vi "Lab Panel V4.91.vi"() -> ()   [LabVIEW 2013] (continued)
                            n840 = call "Save data file (stop) v3.vi"("panel id"=w1524) -> ("network file save error"=w1523:errorcluster)  [unwired: 9 in, 1 out]
                            n841 = local write "RESULT LAB04-1"(FALSE) -> ()
                            n842 = local write "data file error"(w1523) -> ()
                          }
                        }
                        n843 = Bundle(cluster=w1520, "STATUS"="STOP") -> (w1518:T4)  [unwired: 2 in]
                        n844 = local write "DISP LAB04-1"(w1518) -> ()
                      }
                    }
                  }
                  frame True {
                    n845 = local read "SIG LAB04-1"() -> (w1527:T2)
                    n846 = stacked-sequence {
                      seq-local: [w1538 _] -> [_ w1542]
                      tunnel: w1536 -> [_ w1552]
                      tunnel: w1535 -> [_ w1551]
                      tunnel: w1534 -> [_ w1550]
                      tunnel: w1533 -> [_ w1549]
                      tunnel: w1532 -> [_ w1548]
                      tunnel: [_ w1547] -> w1531
                      tunnel: w1530 -> [_ w1546]
                      tunnel: w1529 -> [_ w1545]
                      tunnel: w1528 -> [_ w1544]
                      tunnel: w1527 -> [w1537 w1543]
                      tunnel: w1526 -> [_ w1541]
                      frame #0 {
                        n847 = Unbundle(w1537) -> ("AMPS"=w1540:dbl)  [unwired: 4 out]
                        n848 = call "Check For Amps on v1.vi"("ID"="LAB04-1", "amps"=w1540) -> ("amps"=w1538:bool)  [unwired: 9 in]
                      }
                      frame #1 {
                        n849 = case shown="True" w1542 {
                          tunnel: w1552 -> [_ w1565]
                          tunnel: w1551 -> [_ w1564]
                          tunnel: w1550 -> [_ w1563]
                          tunnel: w1549 -> [_ w1562]
                          tunnel: w1548 -> [_ w1561]
                          tunnel: [errorcluster {"status"=FALSE, "code"=0, "source"=""} ("error out") w1560] -> w1547
                          tunnel: w1546 -> [_ w1559]
                          tunnel: w1545 -> [_ w1558]
                          tunnel: w1544 -> [_ w1557]
                          tunnel: w1543 -> [_ w1556]
                          tunnel: w1541 -> [_ w1555]
                          frame False {
                            w1553 = FALSE
                            n850 = local write "RUN LAB04-1"(w1553) -> ()
                            n851 = local write "run lab04-1"(w1553) -> ()
                          }
                          frame True {
                            n852 = stacked-sequence {
                              seq-local: [w1566 _ _ _ _] -> [_ w1590 _ _ _]
                              tunnel: w1565 -> [w1571 _ _ _ _]
                              tunnel: w1564 -> [w1567 _ _ _ _]
                              tunnel: w1563 -> [w1581 _ _ _ _]
                              tunnel: w1562 -> [w1574 _ _ _ _]
                              tunnel: w1561 -> [w1569 _ _ _ _]
                              tunnel: [_ w1585 _ _ _] -> w1560
                              tunnel: w1559 -> [_ _ _ w1611 _]
                              tunnel: w1558 -> [_ _ _ w1610 _]
                              tunnel: w1557 -> [_ _ _ w1609 _]
                              tunnel: w1556 -> [_ _ _ _ _]
                              tunnel: w1555 -> [_ _ _ _ w1625]
                              frame #0 {
                                w1568 = "\\"
                                n853 = local read "SET LAB04-1"() -> (w1576:T5)
                                n854 = case shown="\"CYCLE TEST\"" w1581 {
                                tunnel: ["L04-1-CHART TEST-" "L04-1-CYCLE TEST-" "L04-1-T-RISE TEST-"] -> w1577
                                frame "CHART TEST", Default {
                                }
                                frame "CYCLE TEST" {
                                }
                                frame "T-RISE TEST" {
                                }
                                }
                                n855 = Unbundle(w1576) -> ("DESCRIPTION"=w1575:string)  [unwired: 4 out]
                                n856 = Concatenate Strings(w1571, "\\", w1569, w1568, w1567, w1568) -> (w1578:string)
                                n857 = String To Path(string=w1578) -> (path=w1580:path)
                                n858 = Concatenate Strings(w1578, w1577, w1575, "-", w1574, ".tdms") -> (w1566:string)
                                n859 = Create Folder(path (use dialog)=w1580) -> (error out=w1579:errorcluster)  [unwired: 2 in, 2 out]
                                n860 = global write "Global 1.vi" "LAB04-1 FILE"(w1566) -> ()
                                n861 = call <vilib>:"Clear Errors.vi"("error in (no error)"=w1579) -> ()  [unwired: 6 in, 1 out]
                              }
                              frame #1 {
                                (unwired) FALSE
                                n862 = String To Path(string=w1590) -> (path=w1586:path)
                                n863 = TDMS Open(6:FALSE, 10:T20."create or replace" ("operation (0:open)"), 11:w1586) -> (0:w1585:errorcluster, 3:→"TDMS LAB04-1":refnum<k34>)  [unwired: 4 in]
                              }
                              frame #2 {
                                n864 = local read "SET LAB04-1"() -> (w1596:T5)
                                n865 = local read "TDMS LAB04-1"() -> (w1607:refnum<k34>)
                                n866 = Build Array("Testers Name", "Description", "Set Test Cycles", "T-Rise minutes", "T-Rise Deg C") -> (w1597:string[])
                                n867 = Unbundle(w1596) -> ("NAME"=w1595:string, "DESCRIPTION"=w1594:string, "CYCLES"=w1593:dbl, "T-RISE mins"=w1592:dbl, "T-RISE deg C"=w1591:dbl)
                                n868 = Number To Decimal String(number=w1593) -> (decimal integer string=w1606:string)  [unwired: 1 in]
                                n869 = Number To Decimal String(number=w1592) -> (decimal integer string=w1605:string)  [unwired: 1 in]
                                n870 = Number To Decimal String(number=w1591) -> (decimal integer string=w1604:string)  [unwired: 1 in]
                                n871 = Build Array(w1595, w1594, w1606, w1605, w1604) -> (w1603:string[])
                                n872 = TDMS Set Properties(5:w1603, 7:w1597, 11:w1607) -> ()  [unwired: 3 in, 4 out]
                              }
                              frame #3 {
                                n873 = local read "DISP LAB04-1"() -> (w1612:T4)
                                n874 = Concatenate Strings("LAB04-1  ", w1611) -> (w1613:string)
                                n875 = Two Button Dialog(message=w1613, 1:w1609, 2:w1610) -> (T button?=w1615:bool)
                                n876 = case shown="True" w1615 {
                                tunnel: w1612 -> [w1622 w1623]
                                tunnel: [w1622 w1623] -> w1619
                                tunnel: [w1621 w1624] -> w1618
                                tunnel: [w1620 w1624] -> w1617
                                frame False {
                                n877 = Unbundle(w1622) -> ("CYCLE"=w1621:dbl, "MINS"=w1620:dbl)  [unwired: 1 out]
                                }
                                frame True {
                                w1624 = 0.0
                                }
                                }
                                n878 = Bundle(cluster=w1619, "CYCLE"=w1618, "MINS"=w1617, "STATUS"="RUN") -> (w1608:T4)
                                n879 = local write "DISP LAB04-1"(w1608) -> ()
                              }
                              frame #4 {
                                n880 = local read "TEMP START LAB04-1"() -> (w1627:cluster{"TL":dbl, "TN":dbl})
                                n881 = Bundle(cluster=w1627, "TL"=w1625, "TN"=w1625) -> (w1626:cluster{"TL":dbl, "TN":dbl})
                                n882 = local write "TEMP START LAB04-1"(w1626) -> ()
                              }
                            }
                          }
                        }
                      }
                    }
                  }
                }
              }
              event "RUN LAB04-2": Value Change {
                n883 = event-data() -> ("NewVal"=w1632:bool)  [unwired: 1 in, 5 out]
                n884 = local write "run lab04-2"(w1632) -> ()
                n885 = case shown="True" w1632 {
                  tunnel: w1638 -> [_ w1676]
                  tunnel: w1637 -> [_ w1675]
                  tunnel: w1635 -> [w1640 w1674]
                  tunnel: w1636 -> [_ w1673]
                  tunnel: w1634 -> [_ w1672]
                  tunnel: [w1639 w1671] -> w1633
                  tunnel: w1631 -> [_ w1670]
                  tunnel: w1630 -> [_ w1669]
                  tunnel: w1629 -> [_ w1668]
                  tunnel: w1628 -> [_ w1666]
                  frame False {
                    # "stop test"
                    n886 = stacked-sequence {
                      tunnel: w1640 -> [w1649 _]
                      tunnel: [w1641 _] -> w1639
                      frame #0 {
                        n887 = local read "DISP LAB04-2"() -> (w1648:T4)
                        n888 = Unbundle(w1648) -> ("CYCLE"=w1646:dbl, "MINS"=w1647:dbl)  [unwired: 1 out]
                        n889 = case shown="\"CYCLE TEST\"" w1649 {
                          tunnel: w1647 -> [_ _ w1656]
                          tunnel: w1646 -> [w1654 w1655 _]
                          tunnel: [w1654 w1655 w1656] -> w1645
                          frame "CHART TEST", Default {
                          }
                          frame "CYCLE TEST" {
                          }
                          frame "T-RISE TEST" {
                          }
                        }
                        n890 = local read "TDMS LAB04-2"() -> (w1653:refnum<k34>)
                        n891 = Build Array("STOPPED") -> (w1650:string[])
                        n892 = Build Array(w1645) -> (w1644:dbl[])
                        n893 = TDMS Write(0:w1653, 5:"TEST RESULT", 7:w1650, 9:w1644) -> (4:w1642:refnum<k34>, 15:w1643:errorcluster)  [unwired: 2 in, 2 out]
                        n894 = TDMS Close(8:w1643, 11:w1642) -> (0:w1641:errorcluster)  [unwired: 1 out]
                      }
                      frame #1 {
                        n895 = local read "DISP LAB04-2"() -> (w1660:T4)
                        n896 = stacked-sequence {
                          tunnel: "LAB04-2" -> [w1662 w1664]
                          frame #0 {
                            n897 = call "sub vi - defrag tdms v1.vi"("panel id"=w1662) -> ("error out"=w1661:errorcluster)  [unwired: 10 in]
                            n898 = local write "data file error"(w1661) -> ()
                          }
                          frame #1 {
                            n899 = call "Save data file (stop) v3.vi"("panel id"=w1664) -> ("network file save error"=w1663:errorcluster)  [unwired: 9 in, 1 out]
                            n900 = local write "RESULT LAB04-2"(FALSE) -> ()
                            n901 = local write "data file error"(w1663) -> ()
                          }
                        }
                        n902 = Bundle(cluster=w1660, "STATUS"="STOP") -> (w1658:T4)  [unwired: 2 in]
                        n903 = local write "DISP LAB04-2"(w1658) -> ()
                      }
                    }
                  }
                  frame True {
                    n904 = local read "SIG LAB04-2"() -> (w1667:T2)
                    n905 = stacked-sequence {
                      seq-local: [w1678 _] -> [_ w1682]
                      tunnel: w1676 -> [_ w1692]
                      tunnel: w1675 -> [_ w1691]
                      tunnel: w1674 -> [_ w1690]
                      tunnel: w1673 -> [_ w1689]
                      tunnel: w1672 -> [_ w1688]
                      tunnel: [_ w1687] -> w1671
                      tunnel: w1670 -> [_ w1686]
                      tunnel: w1669 -> [_ w1685]
                      tunnel: w1668 -> [_ w1684]
                      tunnel: w1667 -> [w1677 w1683]
                      tunnel: w1666 -> [_ w1681]
                      frame #0 {
                        n906 = Unbundle(w1677) -> ("AMPS"=w1680:dbl)  [unwired: 4 out]
                        n907 = call "Check For Amps on v1.vi"("ID"="LAB04-2", "amps"=w1680) -> ("amps"=w1678:bool)  [unwired: 9 in]
                      }
                      frame #1 {
                        n908 = case shown="True" w1682 {
                          tunnel: w1692 -> [_ w1705]
                          tunnel: w1691 -> [_ w1704]
                          tunnel: w1690 -> [_ w1703]
                          tunnel: w1689 -> [_ w1702]
                          tunnel: w1688 -> [_ w1701]
                          tunnel: [errorcluster {"status"=FALSE, "code"=0, "source"=""} ("error out") w1700] -> w1687
                          tunnel: w1686 -> [_ w1699]
                          tunnel: w1685 -> [_ w1698]
                          tunnel: w1684 -> [_ w1697]
                          tunnel: w1683 -> [_ w1696]
                          tunnel: w1681 -> [_ w1695]
                          frame False {
                            w1693 = FALSE
                            n909 = local write "RUN LAB04-2"(w1693) -> ()
                            n910 = local write "run lab04-2"(w1693) -> ()
                          }
                          frame True {
                            n911 = stacked-sequence {
                              seq-local: [w1706 _ _ _ _] -> [_ w1730 _ _ _]
                              tunnel: w1705 -> [w1711 _ _ _ _]
                              tunnel: w1704 -> [w1707 _ _ _ _]
                              tunnel: w1703 -> [w1721 _ _ _ _]
                              tunnel: w1702 -> [w1714 _ _ _ _]
                              tunnel: w1701 -> [w1709 _ _ _ _]
                              tunnel: [_ w1725 _ _ _] -> w1700
                              tunnel: w1699 -> [_ _ _ w1751 _]
                              tunnel: w1698 -> [_ _ _ w1750 _]
                              tunnel: w1697 -> [_ _ _ w1749 _]
                              tunnel: w1696 -> [_ _ _ _ _]
                              tunnel: w1695 -> [_ _ _ _ w1765]
                              frame #0 {
                                w1708 = "\\"
                                n912 = local read "SET LAB04-2"() -> (w1716:T5)
                                n913 = case shown="\"CHART TEST\", Default" w1721 {
                                tunnel: ["L04-2-CHART TEST-" "L04-2-CYCLE TEST-" "L04-2-T-RISE TEST-"] -> w1717
                                frame "CHART TEST", Default {
                                }
                                frame "CYCLE TEST" {
                                }
                                frame "T-RISE TEST" {
                                }
                                }
                                n914 = Unbundle(w1716) -> ("DESCRIPTION"=w1715:string)  [unwired: 4 out]
                                n915 = Concatenate Strings(w1711, "\\", w1709, w1708, w1707, w1708) -> (w1718:string)
                                n916 = String To Path(string=w1718) -> (path=w1720:path)
                                n917 = Concatenate Strings(w1718, w1717, w1715, "-", w1714, ".tdms") -> (w1706:string)
                                n918 = Create Folder(path (use dialog)=w1720) -> (error out=w1719:errorcluster)  [unwired: 2 in, 2 out]
                                n919 = global write "Global 1.vi" "LAB04-2 FILE"(w1706) -> ()
                                n920 = call <vilib>:"Clear Errors.vi"("error in (no error)"=w1719) -> ()  [unwired: 6 in, 1 out]
                              }
                              frame #1 {
                                (unwired) FALSE
                                n921 = String To Path(string=w1730) -> (path=w1726:path)
                                n922 = TDMS Open(6:FALSE, 10:T20."create or replace" ("operation (0:open)"), 11:w1726) -> (0:w1725:errorcluster, 3:→"TDMS LAB04-2":refnum<k34>)  [unwired: 4 in]
                              }
                              frame #2 {
                                n923 = local read "SET LAB04-2"() -> (w1736:T5)
                                n924 = local read "TDMS LAB04-2"() -> (w1747:refnum<k34>)
                                n925 = Build Array("Testers Name", "Description", "Set Test Cycles", "T-Rise minutes", "T-Rise Deg C") -> (w1737:string[])
                                n926 = Unbundle(w1736) -> ("NAME"=w1735:string, "DESCRIPTION"=w1734:string, "CYCLES"=w1733:dbl, "T-RISE mins"=w1732:dbl, "T-RISE deg C"=w1731:dbl)
                                n927 = Number To Decimal String(number=w1733) -> (decimal integer string=w1746:string)  [unwired: 1 in]
                                n928 = Number To Decimal String(number=w1732) -> (decimal integer string=w1745:string)  [unwired: 1 in]
                                n929 = Number To Decimal String(number=w1731) -> (decimal integer string=w1744:string)  [unwired: 1 in]
                                n930 = Build Array(w1735, w1734, w1746, w1745, w1744) -> (w1743:string[])
                                n931 = TDMS Set Properties(5:w1743, 7:w1737, 11:w1747) -> ()  [unwired: 3 in, 4 out]
                              }
                              frame #3 {
                                n932 = local read "DISP LAB04-2"() -> (w1752:T4)
                                n933 = Concatenate Strings("LAB04-2 ", w1751) -> (w1753:string)
                                n934 = Two Button Dialog(message=w1753, 1:w1749, 2:w1750) -> (T button?=w1755:bool)
                                n935 = case shown="True" w1755 {
                                tunnel: w1752 -> [w1762 w1763]
                                tunnel: [w1762 w1763] -> w1759
                                tunnel: [w1761 w1764] -> w1758
                                tunnel: [w1760 w1764] -> w1757
                                frame False {
                                n936 = Unbundle(w1762) -> ("CYCLE"=w1761:dbl, "MINS"=w1760:dbl)  [unwired: 1 out]
                                }
                                frame True {
                                w1764 = 0.0
                                }
                                }
                                n937 = Bundle(cluster=w1759, "CYCLE"=w1758, "MINS"=w1757, "STATUS"="RUN") -> (w1748:T4)
                                n938 = local write "DISP LAB04-2"(w1748) -> ()
                              }
                              frame #4 {
                                n939 = local read "TEMP START LAB04-2"() -> (w1767:cluster{"TL":dbl, "TN":dbl})
                                n940 = Bundle(cluster=w1767, "TL"=w1765, "TN"=w1765) -> (w1766:cluster{"TL":dbl, "TN":dbl})
                                n941 = local write "TEMP START LAB04-2"(w1766) -> ()
                              }
                            }
                          }
                        }
                      }
                    }
                  }
                }
              }
              event "RUN LAB05-1": Value Change {
                n942 = event-data() -> ("NewVal"=w1772:bool)  [unwired: 1 in, 5 out]
                n943 = local write "run lab05-1"(w1772) -> ()
                n944 = case shown="True" w1772 {
                  tunnel: w1778 -> [_ w1816]
                  tunnel: w1777 -> [_ w1815]
                  tunnel: w1775 -> [w1780 w1814]
                  tunnel: w1776 -> [_ w1813]
                  tunnel: w1774 -> [_ w1812]
                  tunnel: [w1779 w1811] -> w1773
                  tunnel: w1771 -> [_ w1810]
                  tunnel: w1770 -> [_ w1809]
                  tunnel: w1769 -> [_ w1808]
                  tunnel: w1768 -> [_ w1806]
                  frame False {
                    # "stop test"
                    n945 = stacked-sequence {
                      tunnel: w1780 -> [w1789 _]
                      tunnel: [w1781 _] -> w1779
                      frame #0 {
                        n946 = local read "DISP LAB05-1"() -> (w1788:T4)
                        n947 = Unbundle(w1788) -> ("CYCLE"=w1786:dbl, "MINS"=w1787:dbl)  [unwired: 1 out]
                        n948 = case shown="\"CYCLE TEST\"" w1789 {
                          tunnel: w1787 -> [_ _ w1796]
                          tunnel: w1786 -> [w1794 w1795 _]
                          tunnel: [w1794 w1795 w1796] -> w1785
                          frame "CHART TEST", Default {
                          }
                          frame "CYCLE TEST" {
                          }
                          frame "T-RISE TEST" {
                          }
                        }
                        n949 = local read "TDMS LAB05-1"() -> (w1793:refnum<k34>)
                        n950 = Build Array("STOPPED") -> (w1790:string[])
                        n951 = Build Array(w1785) -> (w1784:dbl[])
                        n952 = TDMS Write(0:w1793, 5:"TEST RESULT", 7:w1790, 9:w1784) -> (4:w1782:refnum<k34>, 15:w1783:errorcluster)  [unwired: 2 in, 2 out]
                        n953 = TDMS Close(8:w1783, 11:w1782) -> (0:w1781:errorcluster)  [unwired: 1 out]
                      }
                      frame #1 {
                        n954 = local read "DISP LAB05-1"() -> (w1800:T4)
                        n955 = stacked-sequence {
                          tunnel: "LAB05-1" -> [w1802 w1804]
                          frame #0 {
                            n956 = call "sub vi - defrag tdms v1.vi"("panel id"=w1802) -> ("error out"=w1801:errorcluster)  [unwired: 10 in]
                            n957 = local write "data file error"(w1801) -> ()
                          }
                          frame #1 {
                            n958 = call "Save data file (stop) v3.vi"("panel id"=w1804) -> ("network file save error"=w1803:errorcluster)  [unwired: 9 in, 1 out]
                            n959 = local write "RESULT LAB05-1"(FALSE) -> ()
                            n960 = local write "data file error"(w1803) -> ()
                          }
                        }
                        n961 = Bundle(cluster=w1800, "STATUS"="STOP") -> (w1798:T4)  [unwired: 2 in]
                        n962 = local write "DISP LAB05-1"(w1798) -> ()
                      }
                    }
                  }
                  frame True {
                    n963 = local read "SIG LAB05-1"() -> (w1807:T2)
                    n964 = stacked-sequence {
                      seq-local: [w1818 _] -> [_ w1822]
                      tunnel: w1816 -> [_ w1832]
                      tunnel: w1815 -> [_ w1831]
                      tunnel: w1814 -> [_ w1830]
                      tunnel: w1813 -> [_ w1829]
                      tunnel: w1812 -> [_ w1828]
                      tunnel: [_ w1827] -> w1811
                      tunnel: w1810 -> [_ w1826]
                      tunnel: w1809 -> [_ w1825]
                      tunnel: w1808 -> [_ w1824]
                      tunnel: w1807 -> [w1817 w1823]
                      tunnel: w1806 -> [_ w1821]
                      frame #0 {
                        n965 = Unbundle(w1817) -> ("AMPS"=w1820:dbl)  [unwired: 4 out]
                        n966 = call "Check For Amps on v1.vi"("ID"="LAB05-1", "amps"=w1820) -> ("amps"=w1818:bool)  [unwired: 9 in]
                      }
                      frame #1 {
                        n967 = case shown="True" w1822 {
                          tunnel: w1832 -> [_ w1845]
                          tunnel: w1831 -> [_ w1844]
                          tunnel: w1830 -> [_ w1843]
                          tunnel: w1829 -> [_ w1842]
                          tunnel: w1828 -> [_ w1841]
                          tunnel: [errorcluster {"status"=FALSE, "code"=0, "source"=""} ("error out") w1840] -> w1827
                          tunnel: w1826 -> [_ w1839]
                          tunnel: w1825 -> [_ w1838]
                          tunnel: w1824 -> [_ w1837]
                          tunnel: w1823 -> [_ w1836]
                          tunnel: w1821 -> [_ w1835]
                          frame False {
                            w1833 = FALSE
                            n968 = local write "RUN LAB05-1"(w1833) -> ()
                            n969 = local write "run lab05-1"(w1833) -> ()
                          }
                          frame True {
                            n970 = stacked-sequence {
                              seq-local: [w1846 _ _ _ _] -> [_ w1870 _ _ _]
                              tunnel: w1845 -> [w1851 _ _ _ _]
                              tunnel: w1844 -> [w1847 _ _ _ _]
                              tunnel: w1843 -> [w1861 _ _ _ _]
                              tunnel: w1842 -> [w1854 _ _ _ _]
                              tunnel: w1841 -> [w1849 _ _ _ _]
                              tunnel: [_ w1865 _ _ _] -> w1840
                              tunnel: w1839 -> [_ _ _ w1890 _]
                              tunnel: w1838 -> [_ _ _ w1889 _]
                              tunnel: w1837 -> [_ _ _ w1888 _]
                              tunnel: w1836 -> [_ _ _ _ _]
                              tunnel: w1835 -> [_ _ _ _ w1905]
                              frame #0 {
                                w1848 = "\\"
                                n971 = local read "SET LAB05-1"() -> (w1856:T5)
                                n972 = case shown="\"CYCLE TEST\"" w1861 {
                                tunnel: ["L05-1-CHART TEST-" "L05-1-CYCLE TEST-" "L05-1-T-RISE TEST-"] -> w1857
                                frame "CHART TEST", Default {
                                }
                                frame "CYCLE TEST" {
                                }
                                frame "T-RISE TEST" {
                                }
                                }
                                n973 = Unbundle(w1856) -> ("DESCRIPTION"=w1855:string)  [unwired: 4 out]
                                n974 = Concatenate Strings(w1851, "\\", w1849, w1848, w1847, w1848) -> (w1858:string)
                                n975 = String To Path(string=w1858) -> (path=w1860:path)
                                n976 = Concatenate Strings(w1858, w1857, w1855, "-", w1854, ".tdms") -> (w1846:string)
                                n977 = Create Folder(path (use dialog)=w1860) -> (error out=w1859:errorcluster)  [unwired: 2 in, 2 out]
                                n978 = global write "Global 1.vi" "LAB05-1 FILE"(w1846) -> ()
                                n979 = call <vilib>:"Clear Errors.vi"("error in (no error)"=w1859) -> ()  [unwired: 6 in, 1 out]
                              }
                              frame #1 {
                                (unwired) FALSE
                                n980 = String To Path(string=w1870) -> (path=w1866:path)
                                n981 = TDMS Open(6:FALSE, 10:T20."create or replace" ("operation (0:open)"), 11:w1866) -> (0:w1865:errorcluster, 3:→"TDMS LAB05-1":refnum<k34>)  [unwired: 4 in]
                              }
                              frame #2 {
                                n982 = local read "SET LAB05-1"() -> (w1876:T5)
                                n983 = local read "TDMS LAB05-1"() -> (w1887:refnum<k34>)
                                n984 = Build Array("Testers Name", "Description", "Set Test Cycles", "T-Rise minutes", "T-Rise Deg C") -> (w1877:string[])
                                n985 = Unbundle(w1876) -> ("NAME"=w1875:string, "DESCRIPTION"=w1874:string, "CYCLES"=w1873:dbl, "T-RISE mins"=w1872:dbl, "T-RISE deg C"=w1871:dbl)
                                n986 = Number To Decimal String(number=w1873) -> (decimal integer string=w1886:string)  [unwired: 1 in]
                                n987 = Number To Decimal String(number=w1872) -> (decimal integer string=w1885:string)  [unwired: 1 in]
                                n988 = Number To Decimal String(number=w1871) -> (decimal integer string=w1884:string)  [unwired: 1 in]
                                n989 = Build Array(w1875, w1874, w1886, w1885, w1884) -> (w1883:string[])
                                n990 = TDMS Set Properties(5:w1883, 7:w1877, 11:w1887) -> ()  [unwired: 3 in, 4 out]
                              }
                              frame #3 {
                                n991 = local read "DISP LAB05-1"() -> (w1892:T4)
                                n992 = Concatenate Strings("LAB05-1  ", w1890) -> (w1893:string)
                                n993 = Two Button Dialog(message=w1893, 1:w1888, 2:w1889) -> (T button?=w1895:bool)
                                n994 = case shown="True" w1895 {
                                tunnel: w1892 -> [w1902 w1903]
                                tunnel: [w1902 w1903] -> w1899
                                tunnel: [w1901 w1904] -> w1898
                                tunnel: [w1900 w1904] -> w1897
                                frame False {
                                n995 = Unbundle(w1902) -> ("CYCLE"=w1901:dbl, "MINS"=w1900:dbl)  [unwired: 1 out]
                                }
                                frame True {
                                w1904 = 0.0
                                }
                                }
                                n996 = Bundle(cluster=w1899, "CYCLE"=w1898, "MINS"=w1897, "STATUS"="RUN") -> (w1891:T4)
                                n997 = local write "DISP LAB05-1"(w1891) -> ()
                              }
                              frame #4 {
                                n998 = local read "TEMP START LAB05-1"() -> (w1907:cluster{"TL":dbl, "TN":dbl})
                                n999 = Bundle(cluster=w1907, "TL"=w1905, "TN"=w1905) -> (w1906:cluster{"TL":dbl, "TN":dbl})
                                n1000 = local write "TEMP START LAB05-1"(w1906) -> ()
                              }
                            }
                          }
                        }
                      }
                    }
                  }
                }
              }
              event "RUN LAB05-2": Value Change {
                n1001 = event-data() -> ("NewVal"=w1913:bool)  [unwired: 1 in, 5 out]
                n1002 = local read "SIG LAB05-2"() -> (w1909:T2)
                n1003 = case shown="True" w1913 {
                  tunnel: w1919 -> [_ w1957]
                  tunnel: w1918 -> [_ w1956]
                  tunnel: w1916 -> [w1921 w1955]
                  tunnel: w1917 -> [_ w1954]
                  tunnel: w1915 -> [_ w1953]
                  tunnel: [w1920 w1952] -> w1914
                  tunnel: w1912 -> [_ w1951]
                  tunnel: w1911 -> [_ w1950]
                  tunnel: w1910 -> [_ w1949]
                  tunnel: w1909 -> [_ w1948]
                  tunnel: w1908 -> [_ w1947]
                  frame False {
                    # "stop test"
                    n1004 = stacked-sequence {
                      tunnel: w1921 -> [w1930 _]
                      tunnel: [w1922 _] -> w1920
                      frame #0 {
                        n1005 = local read "DISP LAB05-2"() -> (w1929:T4)
                        n1006 = Unbundle(w1929) -> ("CYCLE"=w1927:dbl, "MINS"=w1928:dbl)  [unwired: 1 out]
                        n1007 = case shown="\"CYCLE TEST\"" w1930 {
                          tunnel: w1928 -> [_ _ w1937]
                          tunnel: w1927 -> [w1935 w1936 _]
                          tunnel: [w1935 w1936 w1937] -> w1926
                          frame "CHART TEST", Default {
                          }
                          frame "CYCLE TEST" {
                          }
                          frame "T-RISE TEST" {
                          }
                        }
                        n1008 = local read "TDMS LAB05-2"() -> (w1934:refnum<k34>)
                        n1009 = Build Array("STOPPED") -> (w1931:string[])
                        n1010 = Build Array(w1926) -> (w1925:dbl[])
                        n1011 = TDMS Write(0:w1934, 5:"TEST RESULT", 7:w1931, 9:w1925) -> (4:w1923:refnum<k34>, 15:w1924:errorcluster)  [unwired: 2 in, 2 out]
                        n1012 = TDMS Close(8:w1924, 11:w1923) -> (0:w1922:errorcluster)  [unwired: 1 out]
                      }
                      frame #1 {
                        n1013 = local read "DISP LAB05-2"() -> (w1941:T4)
                        n1014 = stacked-sequence {
                          tunnel: "LAB05-2" -> [w1943 w1945]
                          frame #0 {
                            n1015 = call "sub vi - defrag tdms v1.vi"("panel id"=w1943) -> ("error out"=w1942:errorcluster)  [unwired: 10 in]
                            n1016 = local write "data file error"(w1942) -> ()
                          }
                          frame #1 {
                            n1017 = local write "RESULT LAB05-2"(FALSE) -> ()
                            n1018 = call "Save data file (stop) v3.vi"("panel id"=w1945) -> ("network file save error"=w1944:errorcluster)  [unwired: 9 in, 1 out]
                            n1019 = local write "data file error"(w1944) -> ()
                          }
                        }
                        n1020 = Bundle(cluster=w1941, "STATUS"="STOP") -> (w1939:T4)  [unwired: 2 in]
                        n1021 = local write "DISP LAB05-2"(w1939) -> ()
                      }
                    }
                  }
                  frame True {
                    n1022 = stacked-sequence {
                      seq-local: [w1959 _] -> [_ w1963]
                      tunnel: w1957 -> [_ w1973]
                      tunnel: w1956 -> [_ w1972]
                      tunnel: w1955 -> [_ w1971]
                      tunnel: w1954 -> [_ w1970]
                      tunnel: w1953 -> [_ w1969]
                      tunnel: [_ w1968] -> w1952
                      tunnel: w1951 -> [_ w1967]
                      tunnel: w1950 -> [_ w1966]
                      tunnel: w1949 -> [_ w1965]
                      tunnel: w1948 -> [w1958 w1964]
                      tunnel: w1947 -> [_ w1962]
                      frame #0 {
                        n1023 = Unbundle(w1958) -> ("AMPS"=w1961:dbl)  [unwired: 4 out]
                        n1024 = call "Check For Amps on v1.vi"("ID"="LAB05-2", "amps"=w1961) -> ("amps"=w1959:bool)  [unwired: 9 in]
                      }
                      frame #1 {
                        n1025 = case shown="True" w1963 {
                          tunnel: w1973 -> [_ w1986]
                          tunnel: w1972 -> [_ w1985]
                          tunnel: w1971 -> [_ w1984]
                          tunnel: w1970 -> [_ w1983]
                          tunnel: w1969 -> [_ w1982]
                          tunnel: [errorcluster {"status"=FALSE, "code"=0, "source"=""} ("error out") w1981] -> w1968
                          tunnel: w1967 -> [_ w1980]
                          tunnel: w1966 -> [_ w1979]
                          tunnel: w1965 -> [_ w1978]
                          tunnel: w1964 -> [_ w1977]
                          tunnel: w1962 -> [_ w1976]
                          frame False {
                            w1974 = FALSE
                            n1026 = local write "RUN LAB05-2"(w1974) -> ()
                            n1027 = local write "run lab05-2"(w1974) -> ()
                          }
                          frame True {
                            n1028 = stacked-sequence {
                              seq-local: [w1987 _ _ _ _] -> [_ w2011 _ _ _]
                              tunnel: w1986 -> [w1992 _ _ _ _]
                              tunnel: w1985 -> [w1988 _ _ _ _]
                              tunnel: w1984 -> [w2002 _ _ _ _]
                              tunnel: w1983 -> [w1995 _ _ _ _]
                              tunnel: w1982 -> [w1990 _ _ _ _]
                              tunnel: [_ w2006 _ _ _] -> w1981
                              tunnel: w1980 -> [_ _ _ w2031 _]
                              tunnel: w1979 -> [_ _ _ w2030 _]
                              tunnel: w1978 -> [_ _ _ w2029 _]
                              tunnel: w1977 -> [_ _ _ _ _]
                              tunnel: w1976 -> [_ _ _ _ w2046]
                              frame #0 {
                                w1989 = "\\"
                                n1029 = local read "SET LAB05-2"() -> (w1997:T5)
                                n1030 = case shown="\"CYCLE TEST\"" w2002 {
                                tunnel: ["L05-2-CHART TEST-" "L05-2-CYCLE TEST-" "L05-2-T-RISE TEST-"] -> w1998
                                frame "CHART TEST", Default {
                                }
                                frame "CYCLE TEST" {
                                }
                                frame "T-RISE TEST" {
                                }
                                }
                                n1031 = Unbundle(w1997) -> ("DESCRIPTION"=w1996:string)  [unwired: 4 out]
                                n1032 = Concatenate Strings(w1992, "\\", w1990, w1989, w1988, w1989) -> (w1999:string)
                                n1033 = String To Path(string=w1999) -> (path=w2001:path)
                                n1034 = Concatenate Strings(w1999, w1998, w1996, "-", w1995, ".tdms") -> (w1987:string)
                                n1035 = Create Folder(path (use dialog)=w2001) -> (error out=w2000:errorcluster)  [unwired: 2 in, 2 out]
                                n1036 = global write "Global 1.vi" "LAB05-2 FILE"(w1987) -> ()
                                n1037 = call <vilib>:"Clear Errors.vi"("error in (no error)"=w2000) -> ()  [unwired: 6 in, 1 out]
                              }
                              frame #1 {
                                (unwired) FALSE
                                n1038 = String To Path(string=w2011) -> (path=w2007:path)
                                n1039 = TDMS Open(6:FALSE, 10:T20."create or replace" ("operation (0:open)"), 11:w2007) -> (0:w2006:errorcluster, 3:→"TDMS LAB05-2":refnum<k34>)  [unwired: 4 in]
                              }
                              frame #2 {
                                n1040 = local read "SET LAB05-2"() -> (w2017:T5)
                                n1041 = local read "TDMS LAB05-2"() -> (w2028:refnum<k34>)
                                n1042 = Build Array("Testers Name", "Description", "Set Test Cycles", "T-Rise minutes", "T-Rise Deg C") -> (w2018:string[])
                                n1043 = Unbundle(w2017) -> ("NAME"=w2016:string, "DESCRIPTION"=w2015:string, "CYCLES"=w2014:dbl, "T-RISE mins"=w2013:dbl, "T-RISE deg C"=w2012:dbl)
                                n1044 = Number To Decimal String(number=w2014) -> (decimal integer string=w2027:string)  [unwired: 1 in]
                                n1045 = Number To Decimal String(number=w2013) -> (decimal integer string=w2026:string)  [unwired: 1 in]
                                n1046 = Number To Decimal String(number=w2012) -> (decimal integer string=w2025:string)  [unwired: 1 in]
                                n1047 = Build Array(w2016, w2015, w2027, w2026, w2025) -> (w2024:string[])
                                n1048 = TDMS Set Properties(5:w2024, 7:w2018, 11:w2028) -> ()  [unwired: 3 in, 4 out]
                              }
                              frame #3 {
                                n1049 = local read "DISP LAB05-2"() -> (w2033:T4)
                                n1050 = Concatenate Strings("LAB05-2  ", w2031) -> (w2034:string)
                                n1051 = Two Button Dialog(message=w2034, 1:w2029, 2:w2030) -> (T button?=w2036:bool)
                                n1052 = case shown="True" w2036 {
                                tunnel: w2033 -> [w2043 w2044]
                                tunnel: [w2043 w2044] -> w2040
                                tunnel: [w2042 w2045] -> w2039
                                tunnel: [w2041 w2045] -> w2038
                                frame False {
                                n1053 = Unbundle(w2043) -> ("CYCLE"=w2042:dbl, "MINS"=w2041:dbl)  [unwired: 1 out]
                                }
                                frame True {
                                w2045 = 0.0
                                }
                                }
                                n1054 = Bundle(cluster=w2040, "CYCLE"=w2039, "MINS"=w2038, "STATUS"="RUN") -> (w2032:T4)
                                n1055 = local write "DISP LAB05-2"(w2032) -> ()
                              }
                              frame #4 {
                                n1056 = local read "TEMP START LAB05-2"() -> (w2048:cluster{"TL":dbl, "TN":dbl})
                                n1057 = Bundle(cluster=w2048, "TL"=w2046, "TN"=w2046) -> (w2047:cluster{"TL":dbl, "TN":dbl})
                                n1058 = local write "TEMP START LAB05-2"(w2047) -> ()
                              }
                            }
                          }
                        }
                      }
                    }
                  }
                }
                n1059 = local write "run lab05-2"(w1913) -> ()
              }
            }
            n1060 = local write "data file error"(w617) -> ()
          }
          frame #4 {
            # "check if test cycles reached for cycle tests, if so then test pass"
            n1061 = stacked-sequence {
              tunnel: w2068 -> [_ _ _ _ _ _ _ _ _ _]
              tunnel: w2067 -> [_ _ _ _ _ _ _ _ _ _]
              tunnel: w2066 -> [_ _ _ _ _ _ _ _ _ _]
              tunnel: w2065 -> [_ _ _ _ _ _ _ _ _ _]
              tunnel: w2064 -> [_ _ _ _ _ _ _ _ _ _]
              tunnel: w2063 -> [_ _ _ _ _ _ _ _ _ _]
              tunnel: w2062 -> [_ _ _ _ _ _ _ _ _ _]
              tunnel: w2061 -> [_ _ _ _ _ _ _ _ _ _]
              tunnel: w2060 -> [_ _ _ _ _ _ _ _ _ _]
              tunnel: w2059 -> [_ _ _ _ _ _ _ _ _ _]
              tunnel: w2058 -> [w2074 _ _ _ _ _ _ _ _ _]
              tunnel: w2057 -> [_ w2109 _ _ _ _ _ _ _ _]
              tunnel: w2056 -> [_ _ w2149 _ _ _ _ _ _ _]
              tunnel: w2055 -> [_ _ _ w2189 _ _ _ _ _ _]
              tunnel: w2054 -> [_ _ _ _ w2229 _ _ _ _ _]
              tunnel: w2053 -> [_ _ _ _ _ w2269 _ _ _ _]
              tunnel: w2052 -> [_ _ _ _ _ _ w2309 _ _ _]
              tunnel: w2051 -> [_ _ _ _ _ _ _ w2349 _ _]
              tunnel: w2050 -> [_ _ _ _ _ _ _ _ w2389 _]
              tunnel: w2049 -> [_ _ _ _ _ _ _ _ _ w2429]
              frame #0 {
                # "LAB01-1"
                n1062 = Less?(x=w2074, y=2) -> (x < y?=w2072:bool)
                n1063 = local read "DISP LAB01-1"() -> (w2075:T4)
                n1064 = Unbundle(w2075) -> ("STATUS"=w2069:string)  [unwired: 2 out]
                n1065 = Equal?(x=w2069, y="RUN") -> (x = y?=w2071:bool)
                n1066 = And(x=w2071, y=w2072) -> (x .and. y?=w2070:bool)
                n1067 = case shown="True" w2070 {
                  tunnel: w2075 -> [_ w2080]
                  tunnel: w2074 -> [_ w2084]
                  frame False {
                  }
                  frame True {
                    n1068 = local read "SET LAB01-1"() -> (w2086:T5)
                    n1069 = local read "TDMS LAB01-1"() -> (w2079:refnum<k34>)
                    n1070 = Unbundle(w2086) -> ("CYCLES"=w2077:dbl, "T-RISE mins"=w2083:dbl)  [unwired: 3 out]
                    n1071 = case shown="\"CYCLE TEST\"" w2084 {
                      tunnel: w2083 -> [_ _ w2093]
                      tunnel: [w2088 w2090 w2093] -> w2082
                      tunnel: w2077 -> [w2088 w2090 _]
                      tunnel: ["CHART PASS" "CYCLE PASS" "T-RISE PASS"] -> w2081
                      frame "CHART TEST", Default {
                      }
                      frame "CYCLE TEST" {
                      }
                      frame "T-RISE TEST" {
                      }
                    }
                    n1072 = Unbundle(w2080) -> ("CYCLE"=w2085:dbl)  [unwired: 2 out]
                    n1073 = Increment(x=w2077) -> (x+1=w2078:dbl)
                    n1074 = Greater Or Equal?(x=w2085, y=w2078) -> (x >= y?=w2087:bool)
                    n1075 = case shown="True" w2087 {
                      tunnel: w2082 -> [w2097 _]
                      tunnel: w2081 -> [w2096 _]
                      tunnel: w2080 -> [w2095 _]
                      tunnel: w2079 -> [w2094 _]
                      frame True {
                        n1076 = stacked-sequence {
                          tunnel: w2097 -> [w2101 _]
                          tunnel: w2096 -> [w2099 w2105]
                          tunnel: w2095 -> [_ w2108]
                          tunnel: w2094 -> [w2098 _]
                          frame #0 {
                            n1077 = Build Array(w2099) -> (w2102:string[])
                            n1078 = Build Array(w2101) -> (w2100:dbl[])
                            n1079 = TDMS Write(0:w2098, 5:"TEST PASS", 7:w2102, 9:w2100) -> (15:w2104:errorcluster)  [unwired: 2 in, 3 out]
                            n1080 = local write "data file error"(w2104) -> ()
                          }
                          frame #1 {
                            n1081 = Bundle(cluster=w2108, "STATUS"=w2105) -> (w2106:T4)  [unwired: 2 in]
                            n1082 = local write "RESULT LAB01-1"(TRUE) -> ()
                            n1083 = local write "DISP LAB01-1"(w2106) -> ()
                          }
                        }
                      }
                      frame False {
                      }
                    }
                  }
                }
              }
              frame #1 {
                # "LAB01-2"
                n1084 = Less?(x=w2109, y=2) -> (x < y?=w2112:bool)
                n1085 = local read "DISP LAB01-2"() -> (w2114:T4)
                n1086 = Unbundle(w2114) -> ("STATUS"=w2115:string)  [unwired: 2 out]
                n1087 = Equal?(x=w2115, y="RUN") -> (x = y?=w2111:bool)
                n1088 = And(x=w2111, y=w2112) -> (x .and. y?=w2110:bool)
                n1089 = case shown="True" w2110 {
                  tunnel: w2114 -> [_ w2120]
                  tunnel: w2109 -> [_ w2124]
                  frame False {
                  }
                  frame True {
                    n1090 = local read "SET LAB01-2"() -> (w2126:T5)
                    n1091 = local read "TDMS LAB01-2"() -> (w2119:refnum<k34>)
                    n1092 = Unbundle(w2126) -> ("CYCLES"=w2117:dbl, "T-RISE mins"=w2123:dbl)  [unwired: 3 out]
                    n1093 = case shown="\"T-RISE TEST\"" w2124 {
                      tunnel: w2123 -> [_ _ w2133]
                      tunnel: [w2128 w2130 w2133] -> w2122
                      tunnel: w2117 -> [w2128 w2130 _]
                      tunnel: ["CHART PASS" "CYCLE PASS" "T-RISE PASS"] -> w2121
                      frame "CHART TEST", Default {
                      }
                      frame "CYCLE TEST" {
                      }
                      frame "T-RISE TEST" {
                      }
                    }
                    n1094 = Unbundle(w2120) -> ("CYCLE"=w2125:dbl)  [unwired: 2 out]
                    n1095 = Increment(x=w2117) -> (x+1=w2118:dbl)
                    n1096 = Greater Or Equal?(x=w2125, y=w2118) -> (x >= y?=w2127:bool)
                    n1097 = case shown="True" w2127 {
                      tunnel: w2122 -> [w2137 _]
                      tunnel: w2121 -> [w2136 _]
                      tunnel: w2120 -> [w2135 _]
                      tunnel: w2119 -> [w2134 _]
                      frame True {
                        n1098 = stacked-sequence {
                          tunnel: w2137 -> [w2141 _]
                          tunnel: w2136 -> [w2139 w2145]
                          tunnel: w2135 -> [_ w2148]
                          tunnel: w2134 -> [w2138 _]
                          frame #0 {
                            n1099 = Build Array(w2139) -> (w2142:string[])
                            n1100 = Build Array(w2141) -> (w2140:dbl[])
                            n1101 = TDMS Write(0:w2138, 5:"TEST PASS", 7:w2142, 9:w2140) -> (15:w2144:errorcluster)  [unwired: 2 in, 3 out]
                            n1102 = local write "data file error"(w2144) -> ()
                          }
                          frame #1 {
                            n1103 = Bundle(cluster=w2148, "STATUS"=w2145) -> (w2146:T4)  [unwired: 2 in]
                            n1104 = local write "RESULT LAB01-2"(TRUE) -> ()
                            n1105 = local write "DISP LAB01-2"(w2146) -> ()
                          }
                        }
                      }
                      frame False {
                      }
                    }
                  }
                }
              }
              frame #2 {
                # "LAB02-1"
                n1106 = Less?(x=w2149, y=2) -> (x < y?=w2152:bool)
                n1107 = local read "DISP LAB02-1"() -> (w2154:T4)
                n1108 = Unbundle(w2154) -> ("STATUS"=w2155:string)  [unwired: 2 out]
                n1109 = Equal?(x=w2155, y="RUN") -> (x = y?=w2151:bool)
                n1110 = And(x=w2151, y=w2152) -> (x .and. y?=w2150:bool)
                n1111 = case shown="True" w2150 {
                  tunnel: w2154 -> [_ w2160]
                  tunnel: w2149 -> [_ w2164]
                  frame False {
                  }
                  frame True {
                    n1112 = local read "SET LAB02-1"() -> (w2166:T5)
                    n1113 = local read "TDMS LAB02-1"() -> (w2159:refnum<k34>)
                    n1114 = Unbundle(w2160) -> ("CYCLE"=w2165:dbl)  [unwired: 2 out]
